vi "KE622x -- Get Results Format.vi"(0 "Resource In":refnum<visa-resource-name>, 1 "Check For SCPI Errors? (T)":bool=TRUE, 11 "error in (no error)":errorcluster) -> (4 "Resource Out (dupl)":refnum<visa-resource-name>, 8 "Results Format":T1, 15 "error out":errorcluster)   [LabVIEW 2020, in "Keithley 622x.lvlib"]
doc: "Returns the current setting for the format of measurements sent from the instrument to the PC, either ASCII, Single Precision, or Double Precision."
uses:
  Keithley 622x.lvlib
  Typedefs/KE622x -- Results Format.ctl
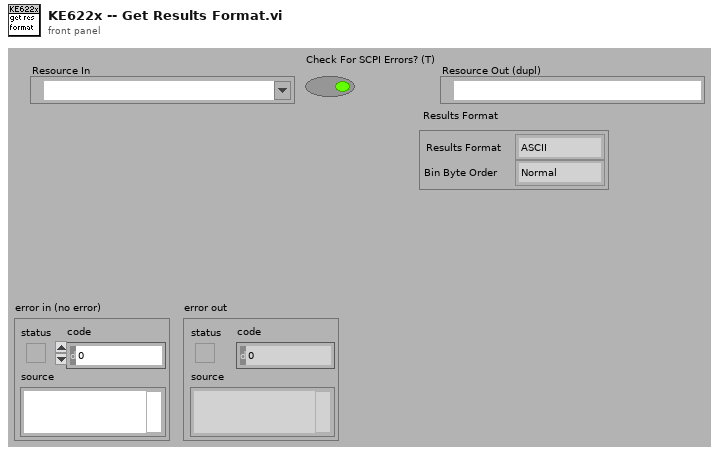
[diagram p1: front panel]
types:
  T1 = typedef "Keithley 622x.lvlib/KE622x -- Results Format.ctl" = cluster{"Results Format":enum16{"ASCII", "Single Prec Bin", "Double Prec Bin"}, "Bin Byte Order":enum16{"Normal", "Swapped"}}
  T2 = enum16{"ASCII", "Single Prec Bin", "Double Prec Bin"}
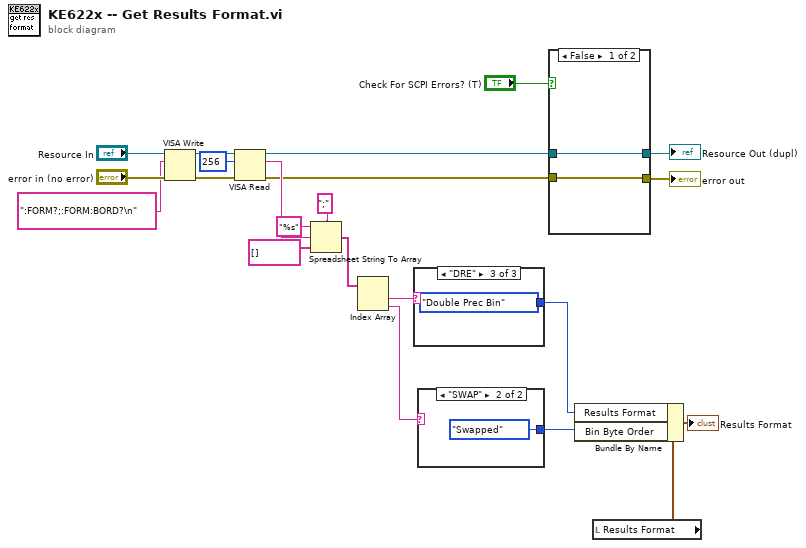
[diagram p0: block diagram]
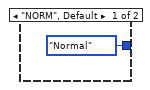
[diagram p2: hidden frame]
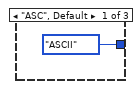
[diagram p3: hidden frame]
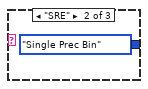
[diagram p4: hidden frame]
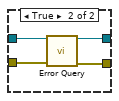
[diagram p5: hidden frame]
diagram:
  n1 = VISA Write(VISA resource name="Resource In", write buffer=":FORM?;:FORM:BORD?\n" ("format string"), error in (no error)="error in (no error)") -> (VISA resource name out=w16:refnum<visa-resource-name>, error out=w15:errorcluster)  [unwired: 1 out]
  n2 = VISA Read(VISA resource name=w16, byte count=u32 256, error in (no error)=w15) -> (VISA resource name out=w13:refnum<visa-resource-name>, read buffer=w10:string, error out=w6:errorcluster)  [unwired: 1 out]
  n3 = Spreadsheet String To Array(delimiter (Tab)=";", format string="%s", spreadsheet string=w10, array type (2D Dbl)=string[] []) -> (array=w5:string[])
  n4 = Index Array(array=w5) -> (element #1=w4:string, element #2=w2:string)  [unwired: 2 in]
  n5 = case shown="\"DRE\"" w4 {
    tunnel: [T2."ASCII" ("Results Format") T2."Single Prec Bin" ("Results Format") T2."Double Prec Bin" ("Results Format")] -> w3
    frame "ASC", Default {
    }
    frame "SRE" {
    }
    frame "DRE" {
    }
  }
  n6 = case shown="\"SWAP\"" w2 {
    tunnel: [enum16{"Normal", "Swapped"}."Normal" ("Bin Byte Order") enum16{"Normal", "Swapped"}."Swapped" ("Bin Byte Order")] -> w1
    frame "NORM", Default {
    }
    frame "SWAP" {
    }
  }
  n7 = case shown="False" "Check For SCPI Errors? (T)" {
    tunnel: w13 -> [w29 w33]
    tunnel: w6 -> [w28 w32]
    tunnel: [w28 w31] -> w18
    tunnel: [w29 w30] -> w19
    frame False {
    }
    frame True {
      n8 = call "Error Query.vi"("VISA Resource In"=w33, "error in (no error)"=w32) -> ("VISA Resource Out (dupl)"=w30:refnum<visa-resource-name>, "error out"=w31:errorcluster)  [unwired: 10 in, 2 out]
    }
  }
  "Resource Out (dupl)" <- w19
  "error out" <- w18
  n9 = local read "Results Format"() -> (w12:T1)
  n10 = Bundle By Name(cluster=w12, "Results Format"=w3, "Bin Byte Order"=w1) -> (→"Results Format":T1)
